vi "initialize vi references.vi"(5 "config class path":path, 7 "runtime class path":path, 8 "error in":errorcluster, 9 "output in":T4, 10 "process in":T5, 11 "input in":T3) -> (0 "error out":errorcluster, 3 "initialized references":T1[](array[typedef]))   [LabVIEW 2013, in "data interface script.lvlib"]
uses:
  data interface script.lvlib
  Controls/processing script control.ctl
  Controls/output script control.ctl
  Controls/input script control.ctl
  Controls/initialized references.ctl
  Controls/interface VI type.ctl
  module/execution/fixed channel runtime.lvclass
  module/configuration/fixed channel configuration.lvclass
  <vilib>/Utility/VariantDataType/VariantType.lvlib
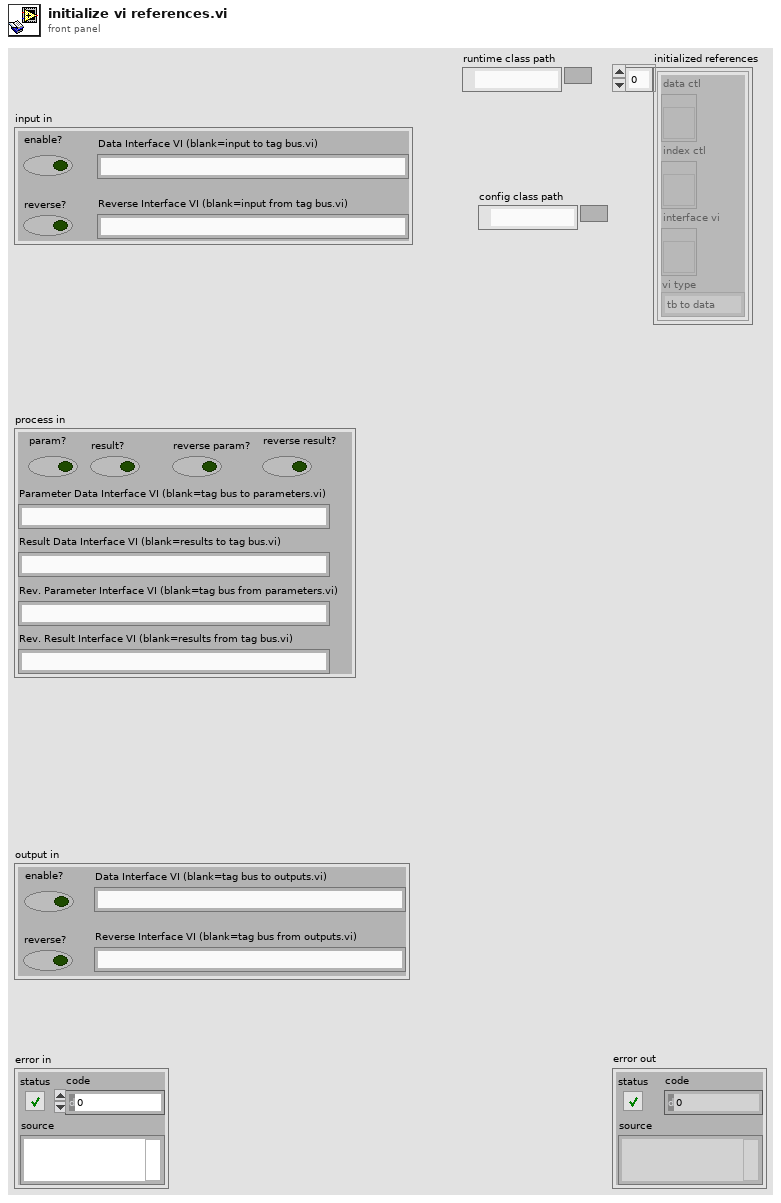
[diagram p1: front panel]
types:
  T1 = typedef "data interface script.lvlib/initialized references.ctl" = cluster{"data ctl":refnum<vi>, "index ctl":refnum<vi>, "interface vi":refnum<vi>, "vi type":T2}
  T2 = typedef "data interface script.lvlib/interface VI type.ctl" = enum16{"tb to data", "data to tb"}
  T3 = typedef "data interface script.lvlib/input script control.ctl" = cluster{"enable?":bool, "Data Interface VI (blank=input to tag bus.vi)":string, "reverse?":bool, "Reverse Interface VI (blank=input from tag bus.vi)":string}
  T4 = typedef "data interface script.lvlib/output script control.ctl" = cluster{"enable?":bool, "Data Interface VI (blank=tag bus to outputs.vi)":string, "Reverse Interface VI (blank=tag bus from outputs.vi)":string, "reverse?":bool}
  T5 = typedef "data interface script.lvlib/processing script control.ctl" = cluster{"param?":bool, "Parameter Data Interface VI (blank=tag bus to parameters.vi)":string, "Result Data Interface VI (blank=results to tag bus.vi)":string, "reverse param?":bool, "Rev. Result Interface VI (blank=results from tag bus.vi)":string, "Rev. Parameter Interface VI (blank=tag bus from parameters.vi)":string, "result?":bool, "reverse result?":bool}
  T6 = typedef "fixed channel runtime.lvclass/data cluster type definition.ctl" = cluster{"input data":variant, "parameter data":variant, "result data":variant, "output data":variant}
  T7 = typedef "fixed channel configuration.lvclass/index type definitions.ctl" = cluster{"input indices":variant, "parameter indices":variant, "result indices":variant, "output indices":variant}
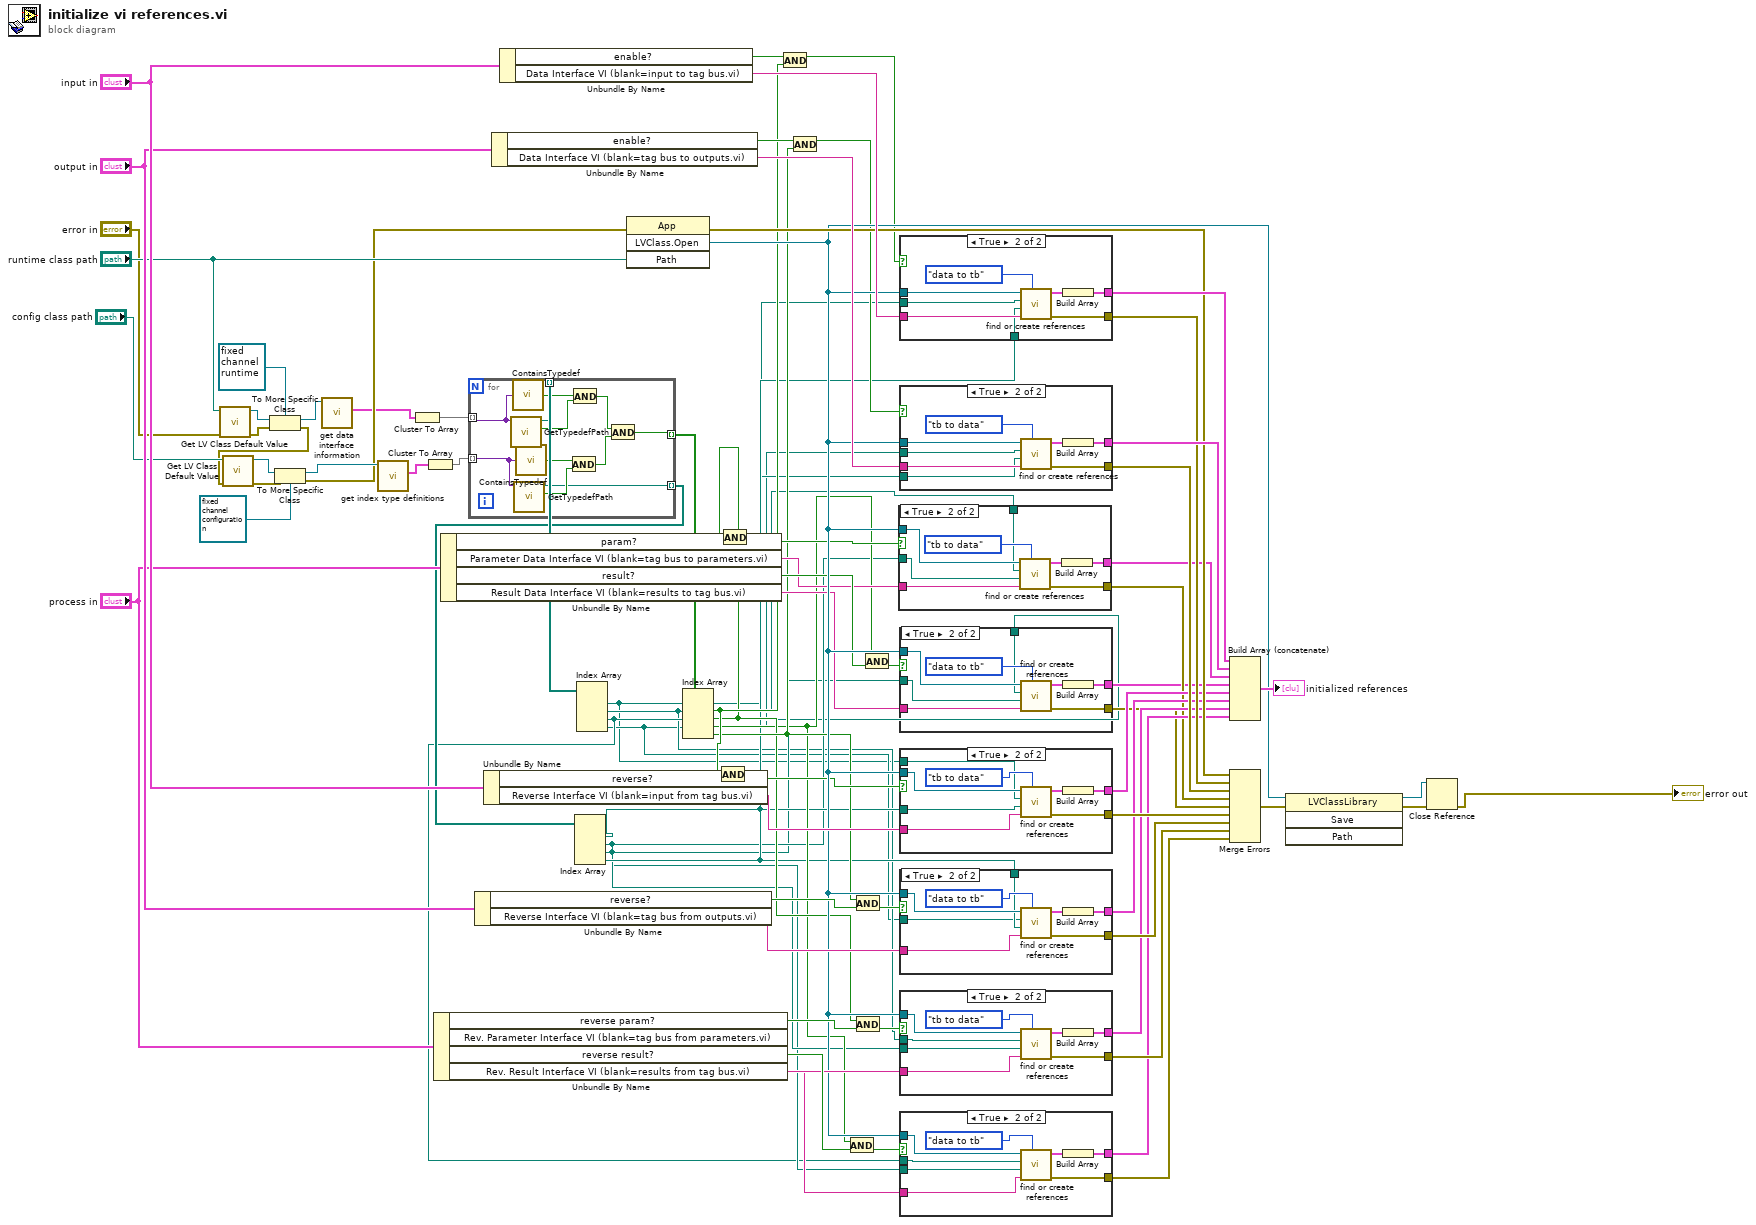
[diagram p0: block diagram]
diagram:
  n1 = call <vilib>:"Get LV Class Default Value.vi"("error in (no error)"="error in", "class path"="runtime class path") -> ("error out"=w37:errorcluster, "object"=w38:refnum<class>)  [unwired: 8 in]
  n2 = To More Specific Class(target class=refnum<class "fixed channel runtime.lvclass"> refnum ("fixed channel runtime"), reference=w38, error in=w37) -> (specific class reference=w34:refnum<class "fixed channel runtime.lvclass">, error out=w32:errorcluster)
  n3 = call <vilib>:"Get LV Class Default Value.vi"("error in (no error)"=w32, "class path"="config class path") -> ("error out"=w40:errorcluster, "object"=w39:refnum<class>)  [unwired: 8 in]
  n4 = To More Specific Class(target class=refnum<class "fixed channel configuration.lvclass"> refnum ("fixed channel configuration"), reference=w39, error in=w40) -> (specific class reference=w33:refnum<class "fixed channel configuration.lvclass">, error out=w31:errorcluster)
  n5 = call-dynamic "get data interface information.vi"("fixed channel runtime in"=w34) -> ("data type defs"=w28:T6)  [unwired: 9 in, 1 out]
  n6 = call-dynamic "get index type definitions.vi"("fixed channel configuration in"=w33) -> ("index type defs"=w29:T7)  [unwired: 9 in, 1 out]
  n7 = Cluster To Array(cluster=w28) -> (array=w26:variant[])
  n8 = Cluster To Array(cluster=w29) -> (array=w27:variant[])
  n9 = Unbundle By Name("process in") -> ("reverse param?"=w53:bool, "Rev. Parameter Interface VI (blank=tag bus from parameters.vi)"=w52:string, "reverse result?"=w54:bool, "Rev. Result Interface VI (blank=results from tag bus.vi)"=w51:string)
  n10 = Unbundle By Name("process in") -> ("param?"=w23:bool, "Parameter Data Interface VI (blank=tag bus to parameters.vi)"=w44:string, "result?"=w45:bool, "Result Data Interface VI (blank=results to tag bus.vi)"=w43:string)
  n11 = for {
    tunnel: w27 -> [w92] mode=indexing
    tunnel: w26 -> [w93] mode=indexing
    tunnel: [w85] -> w16 mode=indexing
    tunnel: [w84] -> w11 mode=indexing
    tunnel: [w83] -> w10 mode=indexing
    n12 = call <vilib>:"GetTypedefPath.vi"("Variant"=w93) -> ("HasPath"=w88:bool, "TypedefPath"=w84:path)  [unwired: 8 in, 1 out]
    n13 = call <vilib>:"ContainsTypedef.vi"("lvvar"=w93) -> ("Contains Typedef"=w89:bool)
    n14 = call <vilib>:"GetTypedefPath.vi"("Variant"=w92) -> ("HasPath"=w90:bool, "TypedefPath"=w83:path)  [unwired: 8 in, 1 out]
    n15 = call <vilib>:"ContainsTypedef.vi"("lvvar"=w92) -> ("Contains Typedef"=w91:bool)
    n16 = And(x=w91, y=w90) -> (x .and. y?=w86:bool)
    n17 = And(x=w89, y=w88) -> (x .and. y?=w87:bool)
    n18 = And(x=w87, y=w86) -> (x .and. y?=w85:bool)
  }
  n19 = Unbundle By Name("output in") -> ("reverse?"=w69:bool, "Reverse Interface VI (blank=tag bus from outputs.vi)"=w68:string)
  n20 = Unbundle By Name("input in") -> ("reverse?"=w66:bool, "Reverse Interface VI (blank=input from tag bus.vi)"=w67:string)
  n21 = Unbundle By Name("output in") -> ("enable?"=w79:bool, "Data Interface VI (blank=tag bus to outputs.vi)"=w80:string)
  n22 = Unbundle By Name("input in") -> ("enable?"=w82:bool, "Data Interface VI (blank=input to tag bus.vi)"=w81:string)
  n23 = Index Array(array=w10) -> (element #1=w9:path, element #2=w7:path, element #3=w6:path, element #4=w8:path)  [unwired: 4 in]
  n24 = Index Array(array=w11) -> (element #1=w2:path, element #2=w4:path, element #3=w5:path, element #4=w3:path)  [unwired: 4 in]
  n25 = invoke class="App" method="LVClass.Open"(error in=w31, "Path"="runtime class path") -> (error out=w72:errorcluster, "LVClass.Open"=w46:refnum<vi>)  [unwired: 2 in, 2 out]
  n26 = Index Array(array=w16) -> (element #1=w15:bool, element #2=w13:bool, element #3=w12:bool, element #4=w14:bool)  [unwired: 4 in]
  n27 = And(x=w15, y=w66) -> (x .and. y?=w20:bool)
  n28 = And(x=w13, y=w23) -> (x .and. y?=w22:bool)
  n29 = And(x=w82, y=w15) -> (x .and. y?=w24:bool)
  n30 = And(x=w79, y=w14) -> (x .and. y?=w25:bool)
  n31 = And(x=w12, y=w54) -> (x .and. y?=w17:bool)
  n32 = And(x=w14, y=w69) -> (x .and. y?=w19:bool)
  n33 = And(x=w13, y=w53) -> (x .and. y?=w18:bool)
  n34 = And(x=w12, y=w45) -> (x .and. y?=w21:bool)
  n35 = case shown="True" w22 {
    tunnel: [_ w100] -> w48
    tunnel: [_ w99] -> w49
    tunnel: w46 -> [_ w97]
    tunnel: w44 -> [_ w96]
    tunnel: w4 -> [_ w95]
    tunnel: w7 -> [_ w94]
    frame False {
    }
    frame True {
      n36 = call "find or create references.vi"("vi type"=interface_VI_type."tb to data", "Data Interface VI"=w96, "index ctl"=w94, "data ctl"=w95, "runtime"=w97) -> ("error out"=w99:errorcluster, "vi refs"=w101:T1)  [unwired: 5 in]
      n37 = Build Array(w101) -> (w100:T1[])
    }
  }
  n38 = case shown="True" w24 {
    tunnel: w81 -> [_ w108]
    tunnel: w46 -> [_ w109]
    tunnel: [_ w106] -> w78
    tunnel: [_ w105] -> w74
    tunnel: w2 -> [_ w103]
    tunnel: w9 -> [_ w102]
    frame False {
    }
    frame True {
      n39 = call "find or create references.vi"("vi type"=interface_VI_type."data to tb", "Data Interface VI"=w108, "index ctl"=w102, "data ctl"=w103, "runtime"=w109) -> ("error out"=w105:errorcluster, "vi refs"=w107:T1)  [unwired: 5 in]
      n40 = Build Array(w107) -> (w106:T1[])
    }
  }
  n41 = case shown="True" w25 {
    tunnel: w80 -> [_ w114]
    tunnel: [_ w116] -> w77
    tunnel: w46 -> [_ w115]
    tunnel: [_ w113] -> w73
    tunnel: w3 -> [_ w111]
    tunnel: w8 -> [_ w110]
    frame False {
    }
    frame True {
      n42 = call "find or create references.vi"("vi type"=interface_VI_type."tb to data", "Data Interface VI"=w114, "index ctl"=w110, "data ctl"=w111, "runtime"=w115) -> ("error out"=w113:errorcluster, "vi refs"=w117:T1)  [unwired: 5 in]
      n43 = Build Array(w117) -> (w116:T1[])
    }
  }
  n44 = case shown="True" w21 {
    tunnel: [_ w124] -> w47
    tunnel: [_ w123] -> w50
    tunnel: w46 -> [_ w121]
    tunnel: w43 -> [_ w120]
    tunnel: w6 -> [_ w119]
    tunnel: w5 -> [_ w118]
    frame False {
    }
    frame True {
      n45 = call "find or create references.vi"("vi type"=interface_VI_type."data to tb", "Data Interface VI"=w120, "index ctl"=w119, "data ctl"=w118, "runtime"=w121) -> ("error out"=w123:errorcluster, "vi refs"=w125:T1)  [unwired: 5 in]
      n46 = Build Array(w125) -> (w124:T1[])
    }
  }
  n47 = case shown="True" w20 {
    tunnel: w67 -> [_ w132]
    tunnel: w46 -> [_ w133]
    tunnel: [_ w130] -> w60
    tunnel: [_ w129] -> w62
    tunnel: w9 -> [_ w127]
    tunnel: w2 -> [_ w126]
    frame False {
    }
    frame True {
      n48 = call "find or create references.vi"("vi type"=interface_VI_type."tb to data", "Data Interface VI"=w132, "index ctl"=w127, "data ctl"=w126, "runtime"=w133) -> ("error out"=w129:errorcluster, "vi refs"=w131:T1)  [unwired: 5 in]
      n49 = Build Array(w131) -> (w130:T1[])
    }
  }
  n50 = case shown="True" w19 {
    tunnel: w68 -> [_ w138]
    tunnel: [_ w140] -> w59
    tunnel: w46 -> [_ w139]
    tunnel: [_ w137] -> w61
    tunnel: w8 -> [_ w135]
    tunnel: w3 -> [_ w134]
    frame False {
    }
    frame True {
      n51 = call "find or create references.vi"("vi type"=interface_VI_type."data to tb", "Data Interface VI"=w138, "index ctl"=w135, "data ctl"=w134, "runtime"=w139) -> ("error out"=w137:errorcluster, "vi refs"=w141:T1)  [unwired: 5 in]
      n52 = Build Array(w141) -> (w140:T1[])
    }
  }
  n53 = case shown="True" w18 {
    tunnel: w52 -> [_ w148]
    tunnel: w46 -> [_ w149]
    tunnel: [_ w146] -> w56
    tunnel: [_ w145] -> w57
    tunnel: w7 -> [_ w143]
    tunnel: w4 -> [_ w142]
    frame False {
    }
    frame True {
      n54 = call "find or create references.vi"("vi type"=interface_VI_type."tb to data", "Data Interface VI"=w148, "index ctl"=w143, "data ctl"=w142, "runtime"=w149) -> ("error out"=w145:errorcluster, "vi refs"=w147:T1)  [unwired: 5 in]
      n55 = Build Array(w147) -> (w146:T1[])
    }
  }
  n56 = case shown="True" w17 {
    tunnel: w51 -> [_ w154]
    tunnel: [_ w156] -> w55
    tunnel: w46 -> [_ w155]
    tunnel: [_ w153] -> w58
    tunnel: w6 -> [_ w151]
    tunnel: w5 -> [_ w150]
    frame False {
    }
    frame True {
      n57 = call "find or create references.vi"("vi type"=interface_VI_type."data to tb", "Data Interface VI"=w154, "index ctl"=w151, "data ctl"=w150, "runtime"=w155) -> ("error out"=w153:errorcluster, "vi refs"=w157:T1)  [unwired: 5 in]
      n58 = Build Array(w157) -> (w156:T1[])
    }
  }
  n59 = Build Array (concatenate)(w78, w77, w48, w47, w60, w59, w56, w55) -> (→"initialized references":T1[])
  n60 = Merge Errors(w72, w74, w73, w49, w50, w62, w61, w57, w58) -> (w76:errorcluster)
  n61 = invoke class="LVClassLibrary" method="Save"(reference=w46, error in=w76) -> (reference out=w70:refnum<vi>, error out=w71:errorcluster)  [unwired: 2 in, 2 out]
  n62 = Close Reference(reference=w70, error in (no error)=w71) -> (error out=→"error out":errorcluster)
